vi "hpcnc try send receive.vi"(8 "error in (no error)":errorcluster, 9 "Max try number":i32, 10 "Send package":string, 11 "VISA Refnum in":refnum<visa-resource-name>) -> (0 "error out":errorcluster, 1 "Receive count":i32, 2 "Receive package":string, 3 "VISA Refnum out":refnum<visa-resource-name>)   [LabVIEW 2014, in "HPCNC.lvlib"]
uses:
  HPCNC.lvlib
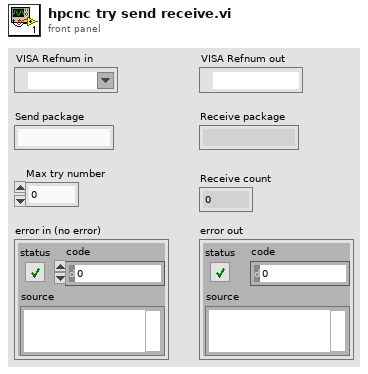
[diagram p1: front panel]
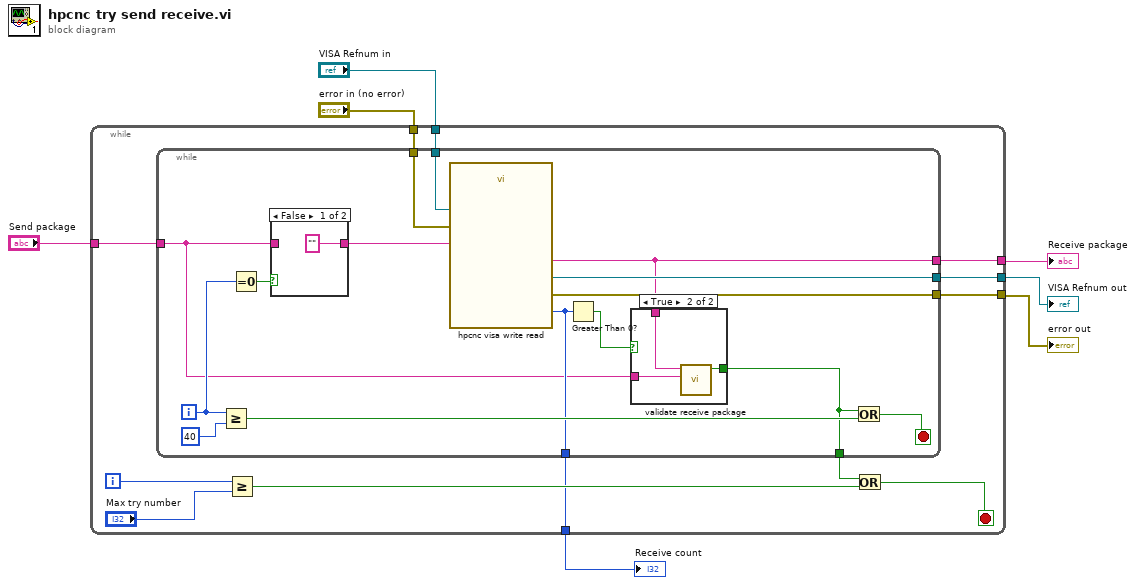
[diagram p0: block diagram]
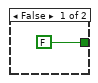
[diagram p2: hidden frame]
diagram:
  n1 = while {
    tunnel: "Send package" -> [w18]
    tunnel: [w14] -> w3
    tunnel: [w13] -> w4
    tunnel: "VISA Refnum in" -> [w12]
    tunnel: "error in (no error)" -> [w11]
    tunnel: [w10] -> w7
    tunnel: [w8] -> w1
    i -> [w19]
    stop <- w15 stop-if-true
    n2 = while {
      tunnel: w18 -> [w21]
      tunnel: [w20] -> w16
      tunnel: [w28] -> w14
      tunnel: [w27] -> w13
      tunnel: w12 -> [w26]
      tunnel: w11 -> [w25]
      tunnel: [w22] -> w10
      tunnel: [w24] -> w8
      i -> [w33]
      stop <- w29 stop-if-true
      n3 = Greater Or Equal?(x=w33, y=40) -> (x >= y?=w30:bool)
      n4 = Equal To 0?(x=w33) -> (x = 0?=w32:bool)
      n5 = case shown="False" w32 {
        tunnel: ["" ("SendData") w40] -> w31
        tunnel: w21 -> [_ w40]
        frame False {
        }
        frame True {
        }
      }
      n6 = call "hpcnc visa write read.vi"("error in (no error)"=w25, "Send data"=w31, "CNC COM in"=w26) -> ("error out"=w28:errorcluster, "Receive buffer"=w22:string, "Receive count"=w24:u32, "CNC COM out"=w27:refnum<visa-resource-name>)  [unwired: 5 in]
      n7 = Greater Than 0?(x=w24) -> (x > 0?=w23:bool)
      n8 = case shown="True" w23 {
        tunnel: w22 -> [_ w38]
        tunnel: w21 -> [_ w37]
        tunnel: [FALSE ("Valid receive package") w36] -> w20
        frame False {
        }
        frame True {
          n9 = call "validate receive package.vi"("Send package"=w37, "Receive package"=w38) -> ("Valid receive package"=w36:bool)  [unwired: 9 in]
        }
      }
      n10 = Or(x=w20, y=w30) -> (x .or. y?=w29:bool)
    }
    n11 = Greater Or Equal?(x=w19, y="Max try number") -> (x >= y?=w17:bool)
    n12 = Or(x=w16, y=w17) -> (x .or. y?=w15:bool)
  }
  "Receive package" <- w7
  "VISA Refnum out" <- w4
  "error out" <- w3
  "Receive count" <- w1
